vi "ClearClipboardData.vi"(8 "No Error":errorcluster) -> (0 "Error Out":errorcluster)   [LabVIEW 2024, in "SDL3.lvlib" / "Clipboard.lvlib"]
doc: "<B>Summary</B>\nClear the clipboard data."
uses:
  Clipboard.lvlib
  Lib/SDL3.dll
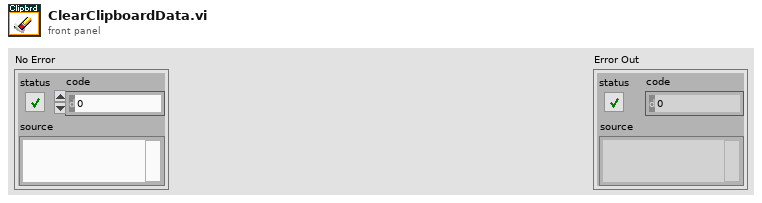
[diagram p1: front panel]
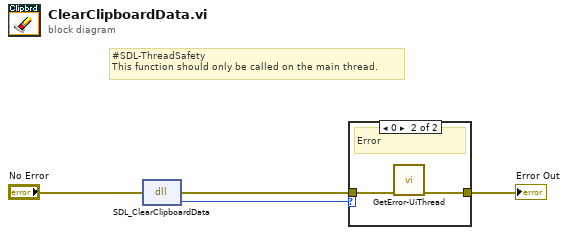
[diagram p0: block diagram]
diagram:
  # "#SDL-ThreadSafety\nThis function should only be called on the main thread."
  n1 = dll-call lib="C:/Users/Thomas/Documents/Projects/LV-SDL3/Sources/SDL3/Lib/SDL3.*" fn="SDL_ClearClipboardData"(error in="No Error") -> (error out=w1:errorcluster, "return type"=w2:i32)  [unwired: 2 in, 1 out]
  n2 = case shown="0" w2 {
    tunnel: w1 -> [w5 w7]
    tunnel: [w5 w6] -> w3
    frame Default {
      # "Ok"
    }
    frame 0 {
      # "Error"
      n3 = call "GetError-UiThread.vi"("No Error"=w7) -> ("error out"=w6:errorcluster)  [unwired: 10 in]
    }
  }
  "Error Out" <- w3
